vi "Name Counter Simple.vi"() -> ()   [LabVIEW 2017]
panel:
  out "Info Sentence":string
  out "Name Sentence":string
  out "Sentence":string
  in  "Name?":bool
  in  "Word":string
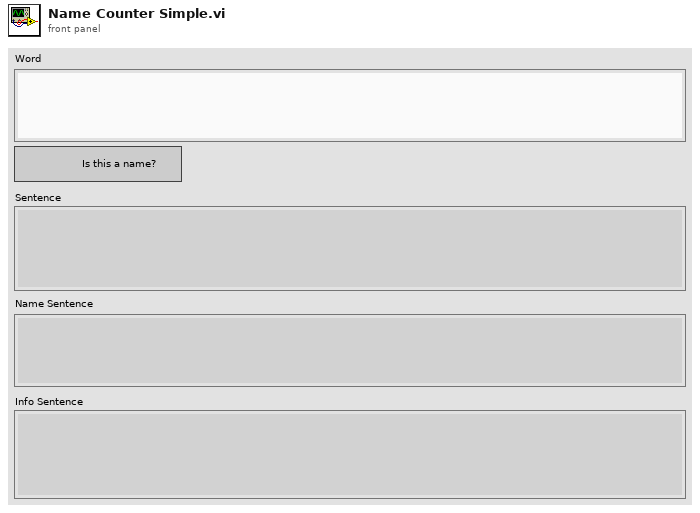
[diagram p1: front panel]
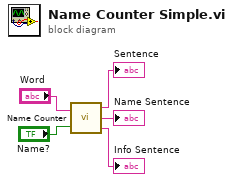
[diagram p0: block diagram]
diagram:
  n1 = call "Name Counter.vi"("Word"="Word", "Name?"="Name?") -> ("Sentence"=→"Sentence":string, "Name Sentence"=→"Name Sentence":string, "Info Sentence"=→"Info Sentence":string)
